vi "destroy.vi"(8 "Error In":errorcluster, 11 "object in":refnum<class "GObject.lvclass">) -> (0 "Error Out":errorcluster)   [LabVIEW 2023, in "TLC_Scripto.lvlib" / "GObject.lvclass"]
uses:
  GObject.lvclass
  GObject.lvclass/GObject.ctl
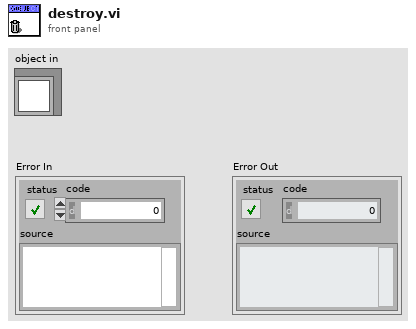
[diagram p1: front panel]
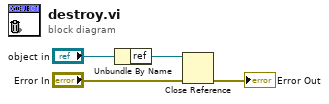
[diagram p0: block diagram]
diagram:
  n1 = Unbundle By Name("object in") -> ("ref"=w3:refnum<vi>)
  n2 = Close Reference(reference=w3, error in (no error)="Error In") -> (error out=→"Error Out":errorcluster)
